vi "Homing.vi"(7 "Model Name":T1, 8 "Error In":errorcluster, 9 "Intialize?":bool=TRUE, 10 "Inputs":T2) -> (0 "error out":errorcluster, 1 "Completed":bool, 4 "Status":cluster{"Status":string, "Elapsed Time":dbl})   [LabVIEW 2017]
doc: "v0.1:\n- Bypass the PES sensor 1 for all front"
uses:
  controls/All Inputs.ctl
  controls/SACB DI.ctl
  controls/Model Name.ctl
  controls/Homing.ctl
  controls/FGV DO.ctl
  GV/All Inputs.vi
panel:
  in  "Delay (for Rest)":u32=500
  in  "Timeout (ms)":u32=15000
  # "Inputs"
  # "Variables"
  # "Outputs"
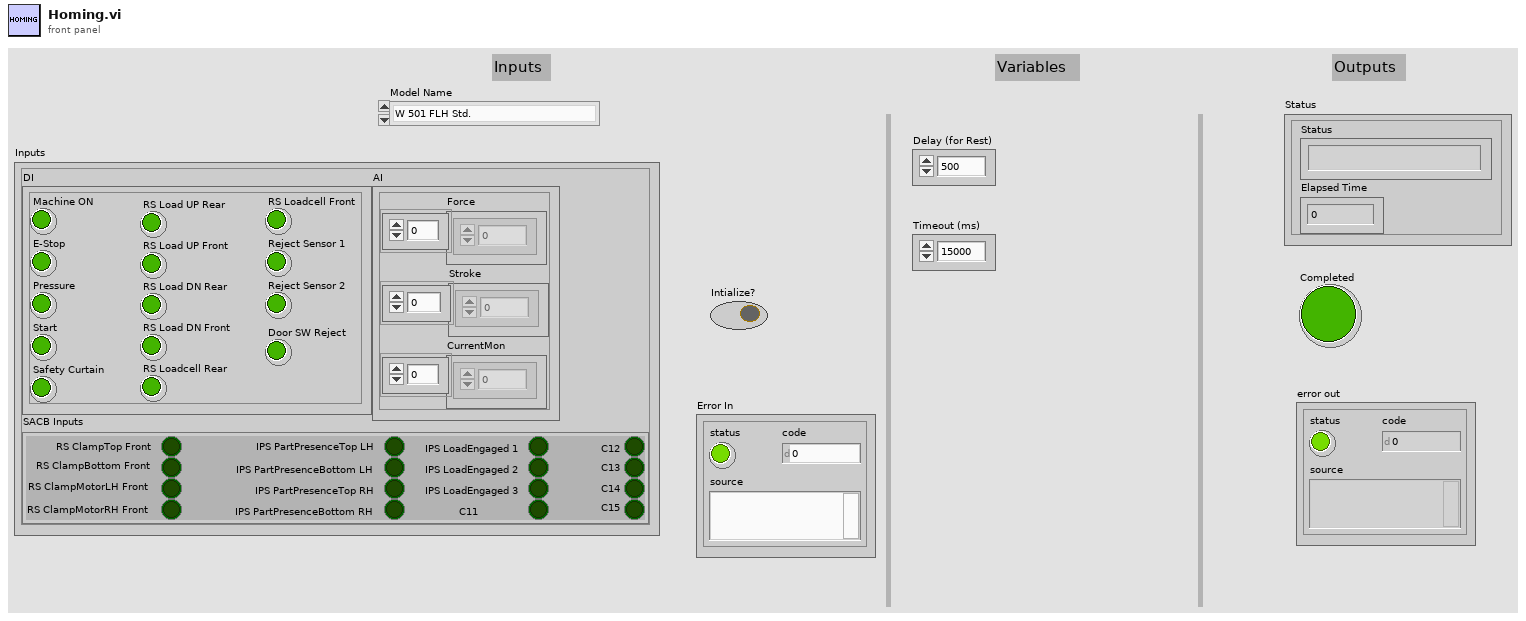
[diagram p1: front panel]
types:
  T1 = typedef "Model Name.ctl" = enum16{"W 501 FLH Std.", "W 501 FRH Std.", "W 601 FR RH Std", "W 601 FR LH Std", "W 601 RR RH Std", "W 601 RR LH Std", "W 601 FR RH AP", "W 601 FR LH AP", "W 601 RR RH AP", "W 601 RR LH AP"}
  T2 = typedef "All Inputs.ctl" = cluster{"DI":cluster{"Machine ON":bool, "E-Stop":bool, "Pressure":bool, "Start":bool, "Safety Curtain":bool, "RS Load UP Rear":bool, "RS Load UP Front":bool, "RS Load DN Rear":bool, "RS Load DN Front":bool, "RS Loadcell Rear":bool, "RS Loadcell Front":bool, "Reject Sensor 1":bool, "Reject Sensor 2":bool, "Door SW Reject":bool}, "AI":cluster{"Force":dbl[], "Stroke":dbl[], "CurrentMon":dbl[]}, "SACB Inputs":T3}
  T3 = typedef "SACB DI.ctl" = cluster{"RS ClampTop Front":bool, "RS ClampBottom Front":bool, "RS ClampMotorLH Front":bool, "RS ClampMotorRH Front":bool, "IPS PartPresenceTop LH":bool, "IPS PartPresenceBottom LH":bool, "IPS PartPresenceTop RH":bool, "IPS PartPresenceBottom RH":bool, "IPS LoadEngaged 1":bool, "IPS LoadEngaged 2":bool, "IPS LoadEngaged 3":bool, "C11":bool, "C12":bool, "C13":bool, "C14":bool, "C15":bool}
  T4 = typedef "Homing.ctl" = enum16{"Initialize", "Loads Disengaged", "Go Down", "Wait for Stall", "Turn Off Supply", "Wait for Rest", "Done", "Error"}
  T5 = typedef "FGV DO.ctl" = enum16{"Initialize", "Start Task", "Clamping", "Load CYL", "Contactors", "Loadcell CYL", "BSL", "Read DO", "Clear Tasks", "Clear Task"}
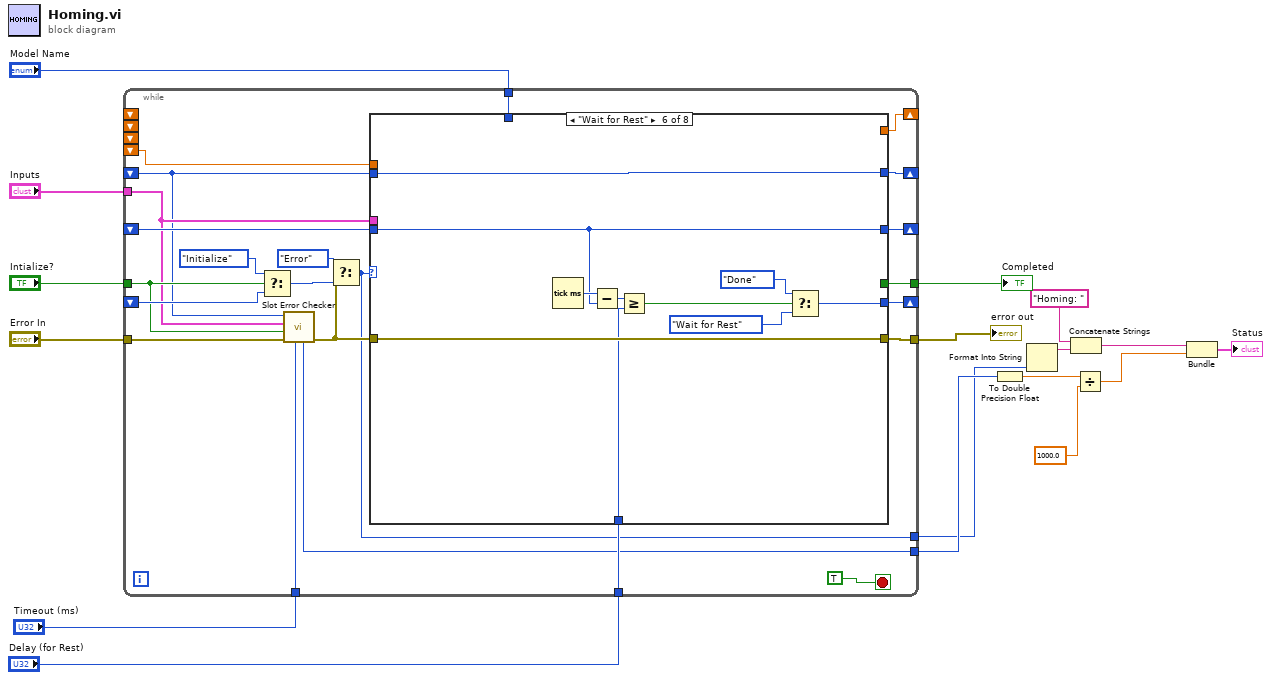
[diagram p0: block diagram]
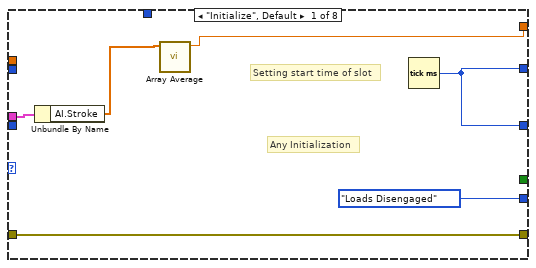
[diagram p2: hidden frame]
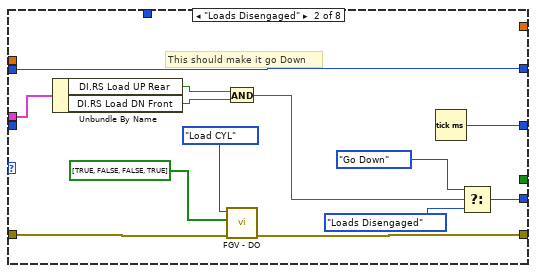
[diagram p3: hidden frame]
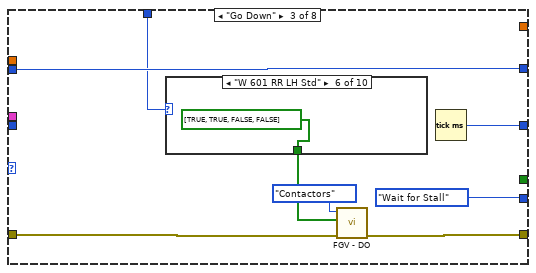
[diagram p4: hidden frame]
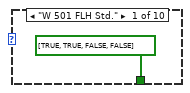
[diagram p5: hidden frame]
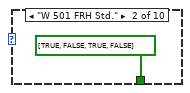
[diagram p6: hidden frame]
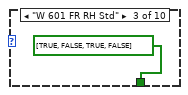
[diagram p7: hidden frame]
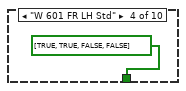
[diagram p8: hidden frame]
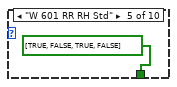
[diagram p9: hidden frame]
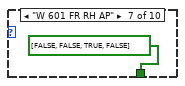
[diagram p10: hidden frame]
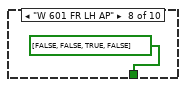
[diagram p11: hidden frame]
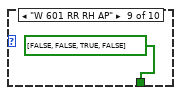
[diagram p12: hidden frame]
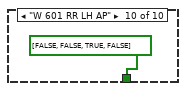
[diagram p13: hidden frame]
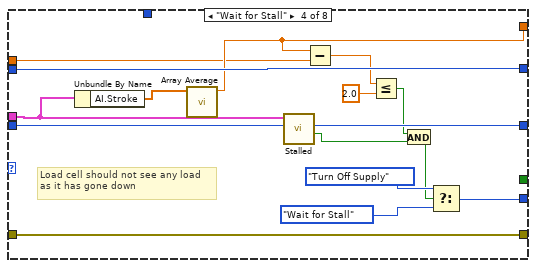
[diagram p14: hidden frame]
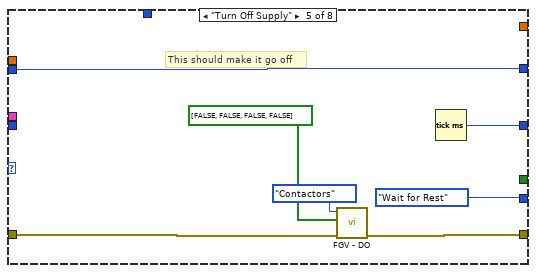
[diagram p15: hidden frame]
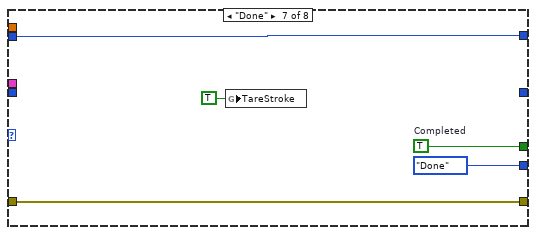
[diagram p16: hidden frame]
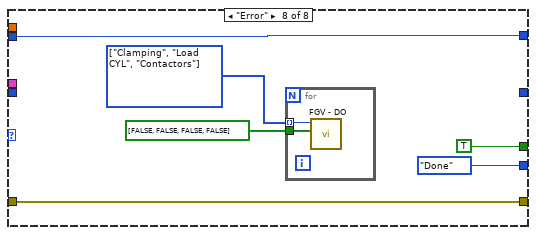
[diagram p17: hidden frame]
diagram:
  n1 = while {
    tunnel: "Intialize?" -> [w30]
    shift-right: [w37] -> _
    shift-left: _ -> [w39]
    shift-right: [w36] -> _
    shift-left: _ -> [w35]
    tunnel: "Error In" -> [w31]
    tunnel: [w34] -> w17
    tunnel: [w33] -> w16
    tunnel: "Inputs" -> [w29]
    shift-right: [w32] -> _
    shift-left: _ -> [w28]
    tunnel: "Delay (for Rest)" -> [w24]
    tunnel: "Timeout (ms)" -> [w23]
    tunnel: "Model Name" -> [w22]
    tunnel: [w21] -> w2
    tunnel: [w20] -> w1
    shift-right: [w19] -> _
    shift-left: _ -> [_]
    shift-left: _ -> [_]
    shift-left: _ -> [_]
    shift-left: _ -> [w18]
    stop <- TRUE stop-if-true
    n2 = Select(t=Homing."Initialize", s=w30, f=w39) -> (s? t:f=w27:T4)
    n3 = call "Slot Error Checker.vi"("Timeout (ms)"=w23, "error in (no error)"=w31, "Intialize?"=w30, "Inputs"=w29, "start time"=w28) -> ("error out"=w26:errorcluster, "Slot Time"=w21:u32)  [unwired: 4 in, 1 out]
    n4 = Select(t=Homing."Error", s=w26, f=w27) -> (s? t:f=w20:T4)
    n5 = case shown="\"Wait for Rest\"" w20 {
      tunnel: [Homing."Loads Disengaged" w52 Homing."Wait for Stall" w87 Homing."Wait for Rest" w107 Homing."Done" Homing."Done"] -> w37
      tunnel: [w44 w55 w62 w90 w95 w109 _ _] -> w36
      tunnel: w35 -> [_ _ _ w91 _ w109 _ _]
      tunnel: w26 -> [w45 w59 w67 w92 w100 w105 w114 w118]
      tunnel: [w45 w58 w66 w92 w99 w105 w114 w118] -> w34
      tunnel: [_ _ _ _ _ _ w113 TRUE ("Completed")] -> w33
      tunnel: w29 -> [w43 w51 _ w86 _ _ _ _]
      tunnel: [w44 w54 w61 w93 w94 w102 w112 w119] -> w32
      tunnel: w28 -> [_ w54 w61 w93 w94 w102 w112 w119]
      tunnel: w24 -> [_ _ _ _ _ w101 _ _]
      tunnel: w22 -> [_ _ w60 _ _ _ _ _]
      tunnel: [w41 _ _ w84 _ _ _ _] -> w19
      tunnel: w18 -> [_ _ _ w83 _ _ _ _]
      frame "Initialize", Default {
        # "Setting start time of slot"
        # "Any Initialization"
        n6 = Unbundle By Name(w43) -> ("AI.Stroke"=w42:dbl[])
        n7 = call "Array Average.vi"("data"=w42) -> ("Numeric"=w41:dbl)  [unwired: 10 in]
        n8 = Tick Count (ms)() -> (millisecond timer value=w44:u32)
      }
      frame "Loads Disengaged" {
        # "This should make it go Down"
        n9 = Unbundle By Name(w51) -> ("DI.RS Load UP Rear"=w50:bool, "DI.RS Load DN Front"=w49:bool)
        n10 = And(x=w50, y=w49) -> (x .and. y?=w47:bool)
        n11 = call "FGV - DO.vi"("error in"=w59, "Digital Outs"=bool[] [TRUE, FALSE, FALSE, TRUE], "State"=FGV_DO."Load CYL") -> ("error out"=w58:errorcluster)  [unwired: 7 in, 1 out]
        n12 = Tick Count (ms)() -> (millisecond timer value=w55:u32)
        n13 = Select(t=Homing."Go Down", s=w47, f=Homing."Loads Disengaged") -> (s? t:f=w52:T4)
      }
      frame "Go Down" {
        n14 = case shown="\"W 601 RR LH Std\"" w60 {
          tunnel: [bool[] [TRUE, TRUE, FALSE, FALSE] ("Digital Outs") bool[] [TRUE, FALSE, TRUE, FALSE] ("Digital Outs") bool[] [TRUE, FALSE, TRUE, FALSE] ("Digital Outs") bool[] [TRUE, TRUE, FALSE, FALSE] ("Digital Outs") bool[] [TRUE, FALSE, TRUE, FALSE] ("Digital Outs") bool[] [TRUE, TRUE, FALSE, FALSE] ("Digital Outs") bool[] [FALSE, FALSE, TRUE, FALSE] ("Digital Outs") bool[] [FALSE, FALSE, TRUE, FALSE] ("Digital Outs") bool[] [FALSE, FALSE, TRUE, FALSE] ("Digital Outs") bool[] [FALSE, FALSE, TRUE, FALSE] ("Digital Outs")] -> w64
          frame "W 501 FLH Std." {
          }
          frame "W 501 FRH Std." {
          }
          frame "W 601 FR RH Std" {
          }
          frame "W 601 FR LH Std" {
          }
          frame "W 601 RR RH Std" {
          }
          frame "W 601 RR LH Std" {
          }
          frame "W 601 FR RH AP" {
          }
          frame "W 601 FR LH AP" {
          }
          frame "W 601 RR RH AP" {
          }
          frame "W 601 RR LH AP" {
          }
        }
        n15 = call "FGV - DO.vi"("error in"=w67, "Digital Outs"=w64, "State"=FGV_DO."Contactors") -> ("error out"=w66:errorcluster)  [unwired: 7 in, 1 out]
        n16 = Tick Count (ms)() -> (millisecond timer value=w62:u32)
      }
      frame "Wait for Stall" {
        # "Load cell should not see any load as it has gone down"
        n17 = Unbundle By Name(w86) -> ("AI.Stroke"=w85:dbl[])
        n18 = call "Array Average.vi"("data"=w85) -> ("Numeric"=w84:dbl)  [unwired: 10 in]
        n19 = call "Stalled.vi"("millisecond timer value in"=w91, "Inputs"=w86) -> ("Stalled"=w79:bool, "millisecond timer value out"=w90:u32)  [unwired: 8 in]
        n20 = Subtract(x=w84, y=w83) -> (x-y=w82:dbl)
        n21 = Less Or Equal?(x=w82, y=2.0) -> (x <= y?=w80:bool)
        n22 = And(x=w80, y=w79) -> (x .and. y?=w78:bool)
        n23 = Select(t=Homing."Turn Off Supply", s=w78, f=Homing."Wait for Stall") -> (s? t:f=w87:T4)
      }
      frame "Turn Off Supply" {
        # "This should make it go off"
        n24 = call "FGV - DO.vi"("error in"=w100, "Digital Outs"=bool[] [FALSE, FALSE, FALSE, FALSE], "State"=FGV_DO."Contactors") -> ("error out"=w99:errorcluster)  [unwired: 7 in, 1 out]
        n25 = Tick Count (ms)() -> (millisecond timer value=w95:u32)
      }
      frame "Wait for Rest" {
        n26 = Tick Count (ms)() -> (millisecond timer value=w110:u32)
        n27 = Subtract(x=w110, y=w109) -> (x-y=w108:u32)
        n28 = Greater Or Equal?(x=w108, y=w101) -> (x >= y?=w106:bool)
        n29 = Select(t=Homing."Done", s=w106, f=Homing."Wait for Rest") -> (s? t:f=w107:T4)
      }
      frame "Done" {
        w113 = TRUE  # Completed
        n30 = global write "All Inputs.vi" "TareStroke"(TRUE ("TareStroke")) -> ()
      }
      frame "Error" {
        w116 = T5[] [enum."Clamping", enum."Load CYL", enum."Contactors"] items=["Initialize", "Start Task", "Clamping", "Load CYL", "Contactors", "Loadcell CYL", "BSL", "Read DO", "Clear Tasks", "Clear Task"]
        n31 = for {
          tunnel: w116 -> [w123] mode=indexing
          tunnel: bool[] [FALSE, FALSE, FALSE, FALSE] ("Digital Outs") -> [w122]
          n32 = call "FGV - DO.vi"("Digital Outs"=w122, "State"=w123) -> ()  [unwired: 8 in, 2 out]
        }
      }
    }
  }
  "error out" <- w17
  "Completed" <- w16
  n33 = To Double Precision Float(number=w2) -> (double precision float=w7:dbl)
  n34 = Format Into String(w1) -> (resulting string=w9:string)  [unwired: 3 in, 1 out]
  n35 = Concatenate Strings("Homing: ", w9) -> (w5:string)
  n36 = Divide(x=w7, y=1000.0) -> (x/y=w4:dbl)
  n37 = Bundle(w5, w4) -> (→"Status":cluster{string, dbl})  [unwired: 1 in]
